vi "Get System Fonts.vi"(3 "error in (no error)":errorcluster) -> (0 "error out":errorcluster, 1 "System Fonts":T1)   [LabVIEW 2013]
doc: "SystemFonts.vi\n\nThis VI reads the windows registry to determine the installed system fonts. Having read the system fonts, the VI filters the font names and assign one to an indicator through a property node.\n\nVersion 1.0\nThis VI is a modified version of \"systemfonts.vi\" which came from Example Program (National Instruments website).\n\nTitle :\"Determining System Fonts and Programmatically Assigning Them to Controls and Indicators\" \n\nLink: http://zone.ni.com/devzone/cda/epd/p/id/1839"
uses:
  Controls/System Fonts.ctl
  <vilib>/registry/registry.llb/Registry RtKey.ctl
  <vilib>/registry/registry.llb/Registry SAM.ctl
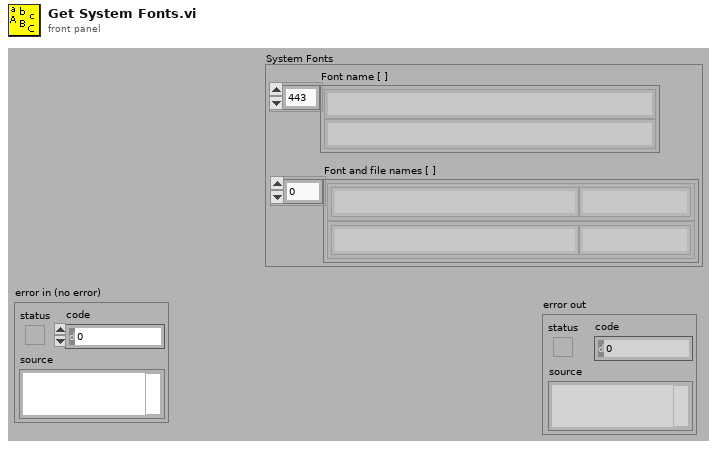
[diagram p1: front panel]
types:
  T1 = typedef "System Fonts.ctl" = cluster{"Font name [ ]":string[], "Font and file names [ ]":cluster{"Font name":string, "File name":string}[]}
  T2 = cluster{"Font name":string, "File name":string}[]
  T3 = typedef "Registry SAM.ctl" = enum32{"KEY_QUERY_VALUE", "KEY_SET_VALUE", "KEY_CREATE_SUB_KEY", "KEY_ENUMERATE_SUB_KEYS", "KEY_NOTIFY", "KEY_CREATE_LINK", "KEY_READ", "KEY_WRITE", "KEY_ALL_ACCESS", "KEY_READ | KEY_WRITE"}
  T4 = typedef "Registry RtKey.ctl" = enum32{"HKEY_CLASSES_ROOT", "HKEY_CURRENT_USER", "HKEY_LOCAL_MACHINE", "HKEY_USERS", "HKEY_PERFORMANCE_DATA", "HKEY_CURRENT_CONFIG", "HKEY_DYN_DATA"}
  T5 = cluster{"value name":string, "string/binary data":string}[]
  T6 = typedef "Registry refnum.ctl" = refnum<k1>
  T7 = cluster{"numValues":i32, "maxValueNameLen":i32, "maxValueDataLen":i32}
  T8 = cluster{"value name":string, "string/binary data":string}
  T9 = cluster{"value name":string, "File name":string}[]
  T10 = cluster{"Font name [ ]":string[], "Font and file names [ ]":cluster{"value name":string, "string/binary data":string}[]}
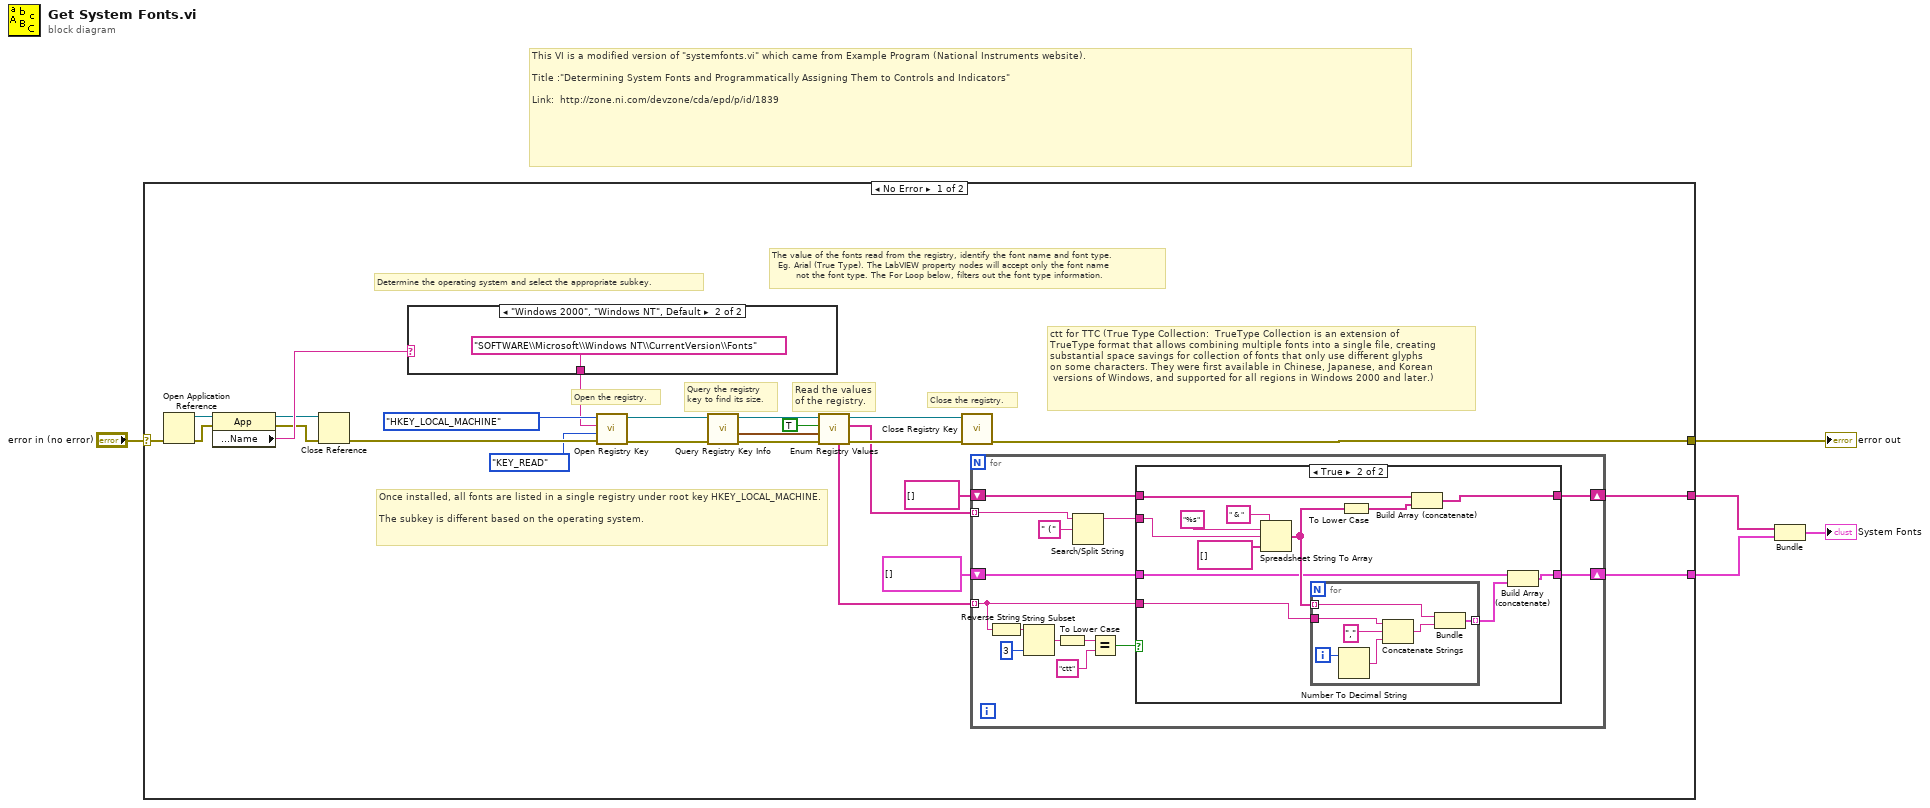
[diagram p0: block diagram]
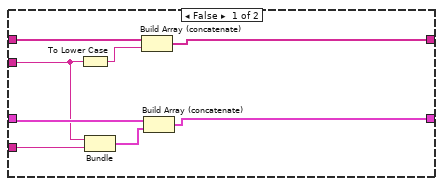
[diagram p2: hidden frame]
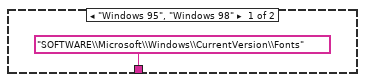
[diagram p3: hidden frame]
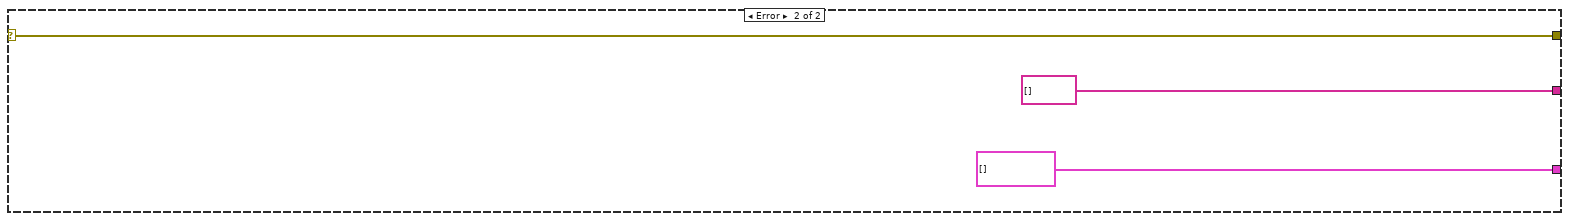
[diagram p4: hidden frame]
diagram:
  # "This VI is a modified version of \"systemfonts.vi\" which came from Example Program (National Instruments website).\n\nTitle :\"Determining System Fonts and Programmatically Assigning Them to Controls and Indicators\" \n\nLink:  http://zone.ni.com/devzone/cda/epd/p/id/1839"
  n1 = case shown="No Error" "error in (no error)" {
    selector: "error in (no error)" -> [w27 w76]
    tunnel: [w28 T5 []] -> w2
    tunnel: [w30 w76] -> w4
    tunnel: [w29 string[] []] -> w3
    frame No Error {
      # "ctt for TTC (True Type Collection:  TrueType Collection is an extension of \nTrueType format that allows combining multiple fonts into a single file, creating\nsubstantial space savings for collection of fonts that only use different glyphs\non some characters. They were first available in Chinese, Japanese, and Korean\n versions of Windows, and supported for all regions in Windows 2000 and later.)"
      # "Determine the operating system and select the appropriate subkey."
      # "The value of the fonts read from the registry, identify the font name and font type. \n  Eg. Arial (True Type). The LabVIEW property nodes will accept only the font name\n        not the font type. The For Loop below, filters out the font type information."
      # "Close the registry."
      # "Query the registry \nkey to find its size."
      # "Open the registry."
      # "Read the values \nof the registry."
      # "Once installed, all fonts are listed in a single registry under root key HKEY_LOCAL_MACHINE.\n\nThe subkey is different based on the operating system."
      n2 = Open Application Reference(8:w27) -> (0:w16:errorcluster, 3:w17:refnum<vi>)  [unwired: 3 out]
      n3 = property class="App"(reference=w17, error in=w16) -> (reference out=w12:refnum<vi>, error out=w13:errorcluster, "Operating System:Name"=w15:string)
      n4 = Close Reference(reference=w12, error in (no error)=w13) -> (error out=w11:errorcluster)
      n5 = case shown="\"Windows 2000\", \"Windows NT\", Default" w15 {
        tunnel: ["SOFTWARE\\Microsoft\\Windows\\CurrentVersion\\Fonts" ("subkey") "SOFTWARE\\Microsoft\\Windows NT\\CurrentVersion\\Fonts" ("subkey")] -> w14
        frame "Windows 95", "Windows 98" {
        }
        frame "Windows 2000", "Windows NT", Default {
        }
      }
      n6 = call <vilib>:"Open Registry Key.vi"("error in (no error)"=w11, "security access mask (KEY_READ | KEY_WRITE)"=Registry_SAM."KEY_READ", "subkey"=w14, "root key (HKEY_LOCAL_MACHINE)"=Registry_RtKey."HKEY_LOCAL_MACHINE") -> ("error out"=w25:errorcluster, "refnum out"=w24:T6)  [unwired: 6 out]
      n7 = call <vilib>:"Query Registry Key Info.vi"("error in (no error)"=w25, "refnum"=w24) -> ("error out"=w21:errorcluster, "value info"=w22:T7, "refnum out"=w23:T6)  [unwired: 7 out]
      n8 = call <vilib>:"Enum Registry Values.vi"("error in (no error)"=w21, "value info"=w22, "retrieve data? (F)"=TRUE, "refnum"=w23) -> ("error out"=w19:errorcluster, "values"=w9:string[], "refnum out"=w20:T6, "String/Binary data"=w8:string[])  [unwired: 1 in, 3 out]
      n9 = call <vilib>:"Close Registry Key.vi"("error in (no error)"=w19, "refnum"=w20) -> ("error out"=w30:errorcluster)  [unwired: 5 out]
      n10 = for {
        tunnel: w9 -> [w43] mode=indexing
        tunnel: w8 -> [w34] mode=indexing
        shift-right: [w35] -> w29
        shift-left: string[] [] ("Font name [ ]") -> [w36]
        shift-right: [w31] -> w28
        shift-left: T2 [] ("Font and file names [ ]") -> [w32]
        n11 = Reverse String(1:w34) -> (0:w42:string)
        n12 = String Subset(string=w42, length (rest)=3 ("length (rest)")) -> (substring=w40:string)  [unwired: 1 out]
        n13 = To Lower Case(string=w40) -> (all lower case string=w38:string)
        n14 = Search/Split String(string=w43, search string/char (-)=" (") -> (substring before match=w33:string)  [unwired: 3 out]
        n15 = Equal?(x=w38, y="ctt") -> (x = y?=w37:bool)
        n16 = case shown="True" w37 {
          tunnel: w36 -> [w52 w61]
          tunnel: [w51 w59] -> w35
          tunnel: w34 -> [w50 w57]
          tunnel: w33 -> [w46 w62]
          tunnel: w32 -> [w49 w56]
          tunnel: [w47 w54] -> w31
          frame False {
            n17 = To Lower Case(string=w46) -> (all lower case string=w45:string)
            n18 = Bundle("value name"=w46, "string/binary data"=w50) -> (w48:T8)  [unwired: 1 out]
            n19 = Build Array (concatenate)(w52, w45) -> (w51:string[])
            n20 = Build Array (concatenate)(w49, w48) -> (w47:T5)
          }
          frame True {
            n21 = Spreadsheet String To Array(delimiter (Tab)=" & ", format string="%s", spreadsheet string=w62, array type (2D Dbl)=string[] [] ("Font name [ ]")) -> (array=w58:string[])
            n22 = for {
              tunnel: w58 -> [w66] mode=indexing
              tunnel: w57 -> [w69]
              tunnel: [w65] -> w55 mode=indexing
              i -> [w71]
              n23 = Number To Decimal String(number=w71) -> (decimal integer string=w70:string)  [unwired: 1 out]
              n24 = Concatenate Strings(w69, ",", w70) -> (w67:string)
              n25 = Bundle("value name"=w66, w67) -> (w65:cluster{"value name":string, string})  [unwired: 1 out]
            }
            n26 = To Lower Case(string=w58) -> (all lower case string=w60:string[])
            n27 = Build Array (concatenate)(w61, w60) -> (w59:string[])
            n28 = Build Array (concatenate)(w56, w55) -> (w54:T9)
          }
        }
      }
    }
    frame Error {
    }
  }
  "error out" <- w4
  n29 = Bundle("Font name [ ]"=w3, "Font and file names [ ]"=w2) -> (→"System Fonts":T10)  [unwired: 1 out]
